vi "Load JSON.vi"(6 "Expand all?":bool, 8 "Error In":errorcluster, 9 "JSON Schema in":string, 10 "<JSON> in":string, 11 "WebView.JSONEditor in":refnum<class "WebView.JSONEditor.lvclass">) -> (0 "Error Out":errorcluster, 3 "WebView.JSONEditor out":refnum<class "WebView.JSONEditor.lvclass">)   [LabVIEW 2024, in "WebView.JSONEditor.lvclass"]
uses:
  WebView.JSONEditor.lvclass
  C:/Git/WebView-Components/WebView_class/WebView.lvclass
  WebView_class/Editor Mode--enum.ctl
  40ff2670-f8ea-4d41-9900-15e563433872.vi
  <vilib>/JDP Science/JSONtext/Variant to JSON Text.vi
  <vilib>/JDP Science/JSONtext/LVClass Serializer/JSONtext LVClass Serializer.lvclass
  WebView_class/WebView.lvclass
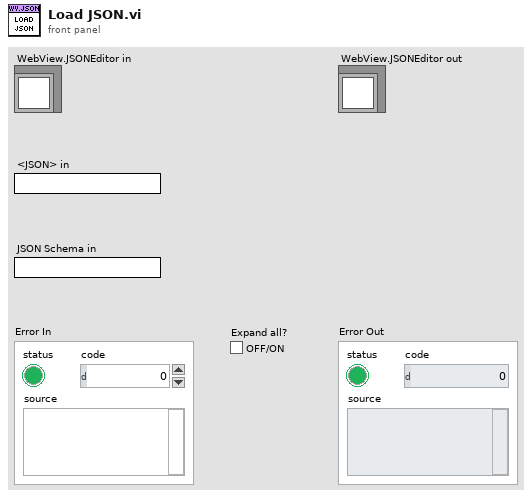
[diagram p1: front panel]
types:
  T1 = typedef "WebView.JSONEditor.lvclass/Editor Mode--enum.ctl" = enum16{"Tree", "View", "Form", "Code", "Text"}
  T2 = cluster{"type":enum16{"loadJSON", "setMode", "getJSON"}, "json":string, "schema":string, "Mode":T1, "expandAll":bool}
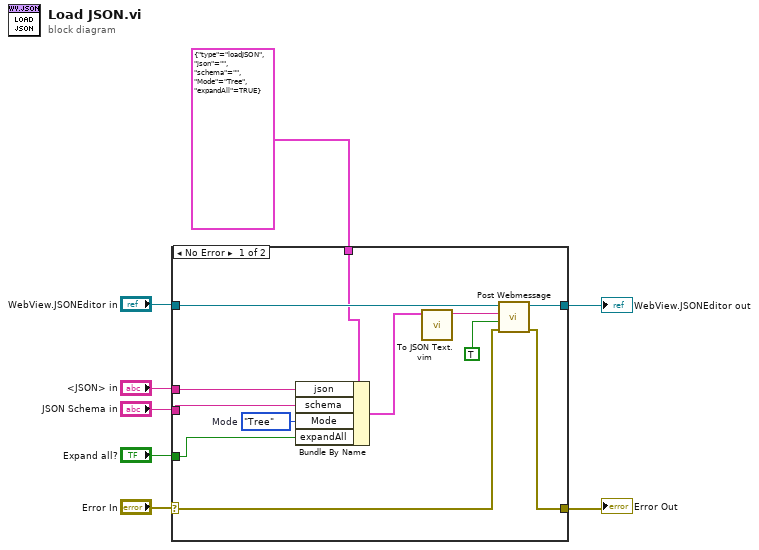
[diagram p0: block diagram]
diagram:
  n1 = case shown="No Error" "Error In" {
    selector: "Error In" -> [w18 w22]
    tunnel: [w17 w22] -> w7
    tunnel: [w16 w21] -> w5
    tunnel: "WebView.JSONEditor in" -> [w20 w21]
    tunnel: "Expand all?" -> [w11 _]
    tunnel: "JSON Schema in" -> [w13 _]
    tunnel: "<JSON> in" -> [w14 _]
    tunnel: T2 {"type"=enum."loadJSON", "json"="", "schema"="", "Mode"=enum."Tree", "expandAll"=TRUE} -> [w15 _]
    frame No Error {
      w12 = Editor_Mode--enum."Tree"  # Mode
      n2 = Bundle By Name(cluster=w15, "json"=w14, "schema"=w13, "Mode"=w12, "expandAll"=w11) -> (w10:T2)
      n3 = call "To JSON Text.vim"("Anything"=w10) -> ("<JSON>"=w9:string)  [unwired: 9 in, 1 out]
      n4 = call "Post Webmessage.vi"("Error In"=w18, "Send as JSON"=TRUE ("Fetch Result? (T)"), "Message"=w9, "WebView in"=w20) -> ("Error Out"=w17:errorcluster, "WebView out"=w16:refnum<class "WebView.JSONEditor.lvclass">)  [unwired: 6 in]
    }
    frame Error {
    }
  }
  "Error Out" <- w7
  "WebView.JSONEditor out" <- w5
